vi "Remember Template info.vi"(10 "Template File":path) -> (0 "Source":string[][](array[string]), 1 "2D Template info":string[][](array[string]), 2 "Ignore":string[][](array[string]), 3 "Maths":string[](array[string]), 5 "Template Ch Names Out":string[](array[string]))   [LabVIEW 2022 SP3]
uses:
  Anemometry/Anemometry Sub Vis/Controls/Global_mode.ctl
  Anemometry/Anemometry Sub Vis/Data_plotting_vis/Results_plotter_Global.vi
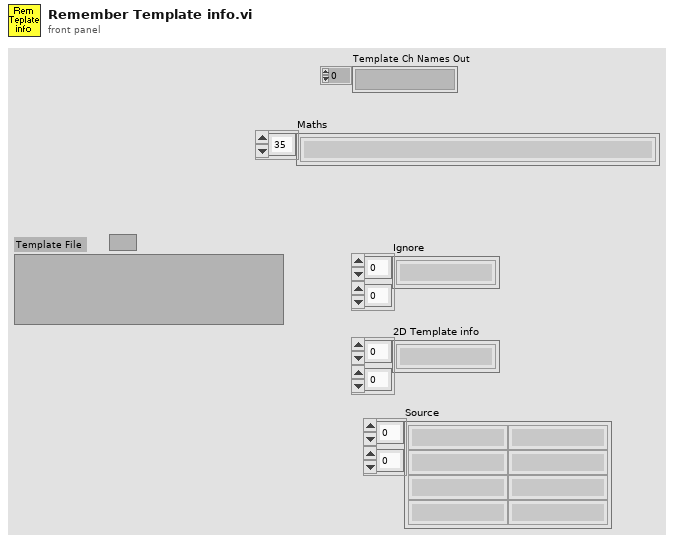
[diagram p1: front panel]
types:
  T1 = typedef "Global_mode.ctl" = enum16{"Read Global", "Load Global From File", "Write Global to File"}
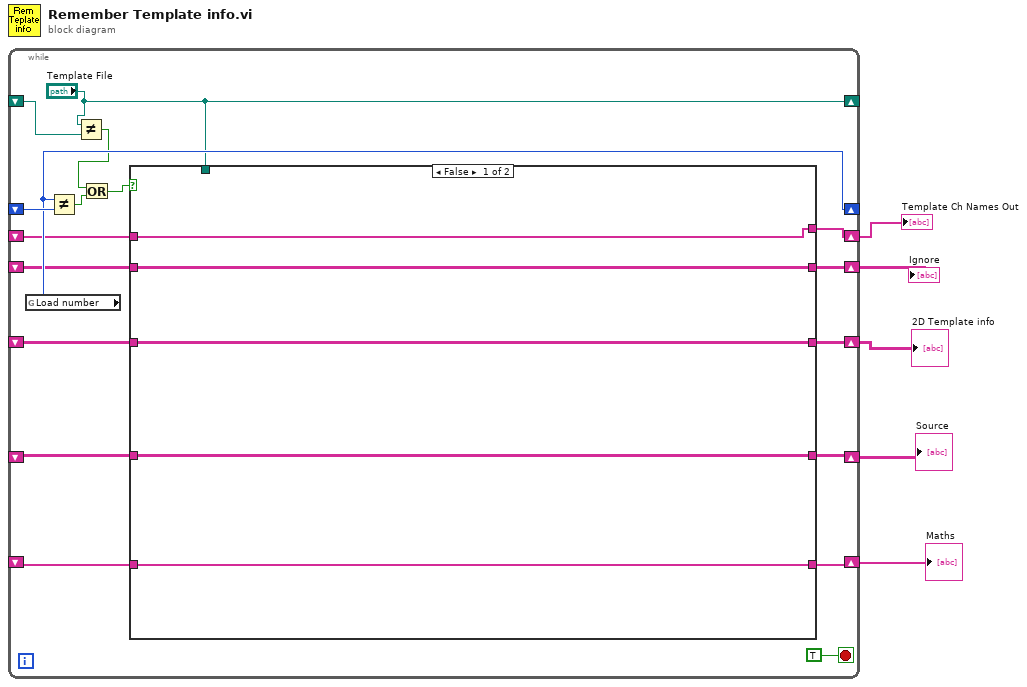
[diagram p0: block diagram]
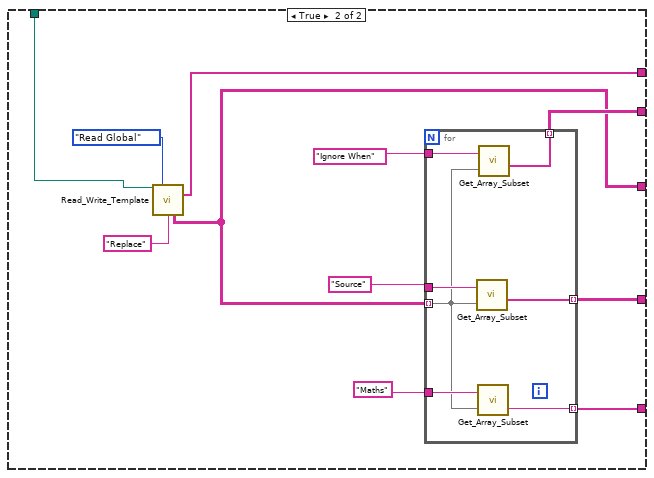
[diagram p2: hidden frame]
diagram:
  n1 = while {
    shift-right: [w19] -> w5
    shift-left: _ -> [w13]
    shift-right: [w20] -> w4
    shift-left: _ -> [w14]
    shift-right: [w21] -> w3
    shift-left: _ -> [w15]
    shift-right: [w22] -> w2
    shift-left: _ -> [w16]
    shift-right: [w17] -> _
    shift-left: _ -> [w18]
    shift-right: [w12] -> w1
    shift-left: _ -> [w11]
    shift-right: ["Template File"] -> _
    shift-left: _ -> [w7]
    stop <- TRUE stop-if-true
    n2 = global read "Results_plotter_Global.vi" "Load number"() -> (w17:i32)
    n3 = Not Equal?(x=w17, y=w18) -> (x != y?=w10:bool)
    n4 = Not Equal?(x="Template File", y=w7) -> (x != y?=w6:bool)
    n5 = Or(x=w6, y=w10) -> (x .or. y?=w9:bool)
    n6 = case shown="False" w9 {
      tunnel: [w28 w34] -> w22
      tunnel: [w27 w30] -> w21
      tunnel: [w26 w33] -> w20
      tunnel: [w25 w32] -> w19
      tunnel: w16 -> [w28 _]
      tunnel: w15 -> [w27 _]
      tunnel: w14 -> [w26 _]
      tunnel: w13 -> [w25 _]
      tunnel: [w24 w31] -> w12
      tunnel: w11 -> [w24 _]
      tunnel: "Template File" -> [_ w29]
      frame False {
      }
      frame True {
        n7 = call "Read_Write_Template.vi"("Template File"=w29, "Mode"=Global_mode."Read Global", "Data type"="Replace") -> ("Template Ch Names Out"=w31:string[], "Template Info"=w30:string[][])  [unwired: 5 in, 6 out]
        n8 = for {
          tunnel: w30 -> [w41] mode=indexing
          tunnel: "Source" -> [w46]
          tunnel: "Maths" -> [w45]
          tunnel: [w44] -> w33 mode=indexing
          tunnel: [w43] -> w32 mode=indexing
          tunnel: "Ignore When" -> [w42]
          tunnel: [w40] -> w34 mode=indexing
          n9 = call "Get_Array_Subset.vi"("String Array In"=w41, "Subset Name"=w46) -> ("Array Subset Out"=w44:string[])  [unwired: 4 out]
          n10 = call "Get_Array_Subset.vi"("String Array In"=w41, "Subset Name"=w45) -> ("First Element"=w43:string)  [unwired: 4 out]
          n11 = call "Get_Array_Subset.vi"("String Array In"=w41, "Subset Name"=w42) -> ("Array Subset Out"=w40:string[])  [unwired: 4 out]
        }
      }
    }
  }
  "Ignore" <- w2
  "2D Template info" <- w3
  "Source" <- w4
  "Maths" <- w5
  "Template Ch Names Out" <- w1
